vi "Tell Self.vi"(4 "Priority":bool, 7 "Actor in":refnum<class "Actor.lvclass">) -> (0 "Error out":errorcluster)   [LabVIEW 2025, in "_Template.lvlib" / "Templates.lvlib" / "TEMPLATE Msg.lvlib"]
uses:
  TEMPLATE Msg.lvlib
  TEMPLATE Msg/TEMPLATE Msg.lvclass
  jettl/jettl/Actor/Actor/Actor.lvclass
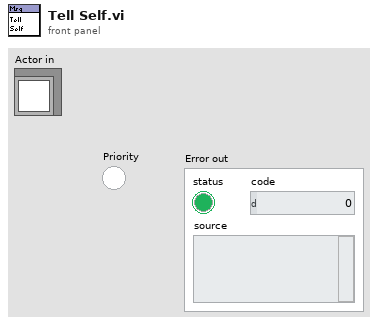
[diagram p1: front panel]
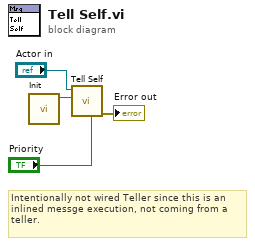
[diagram p0: block diagram]
diagram:
  # "Intentionally not wired Teller since this is an inlined messge execution, not coming from a teller."
  n1 = call "Init.vi"() -> ("TEMPLATE Msg out"=w3:refnum<class "TEMPLATE Msg.lvclass">)  [unwired: 11 in]
  n2 = call-dynamic "Tell Self.vi"("Is Priority"="Priority", "Msg"=w3, "Actor in"="Actor in") -> ("Error out"=→"Error out":errorcluster)  [unwired: 8 in]
